vi "Do transition DSP402.vi"(4 "error in (no error)":errorcluster, 6 "State":T1, 7 "DSP402 in":refnum<class "DSP402.lvclass">) -> (0 "error out":errorcluster, 3 "DSP402 out":refnum<class "DSP402.lvclass">)   [LabVIEW 2017, in "canopen.lvlib" / "DSP402.lvclass"]
uses:
  DSP402.lvclass
  DriveState.ctl
  DSP402.lvclass/DSP402.ctl
  types/threestateFlag.ctl
  canopen.lvlib
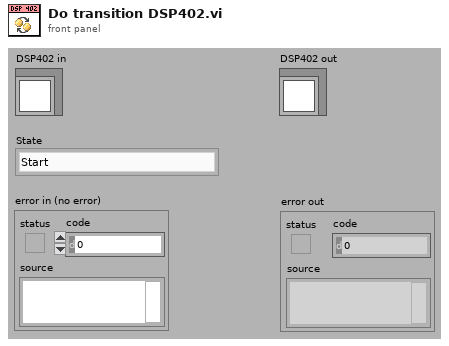
[diagram p1: front panel]
types:
  T1 = typedef "canopen.lvlib/DSP402.lvclass/DriveState.ctl" = enum16{"Start", "Not ready to switch on", "Switch on disabled", "Ready to switch on", "Switched on", "Operation enable", "Fault reaction active", "Fault", "Quick stop active"}
  T2 = typedef "canopen.lvlib/threestateFlag.ctl" = i8
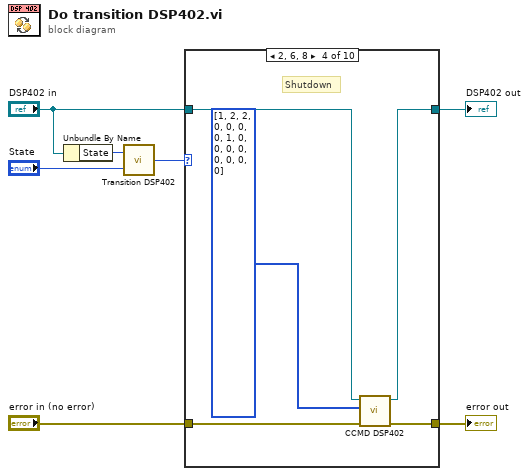
[diagram p0: block diagram]
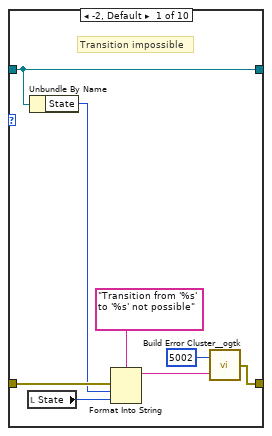
[diagram p2: hidden frame]
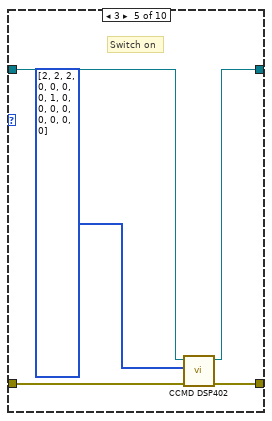
[diagram p5: hidden frame]
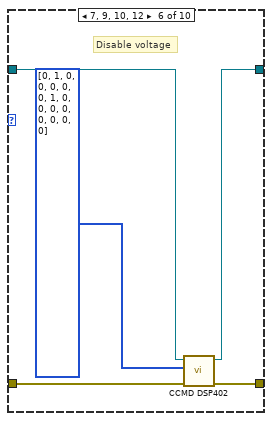
[diagram p6: hidden frame]
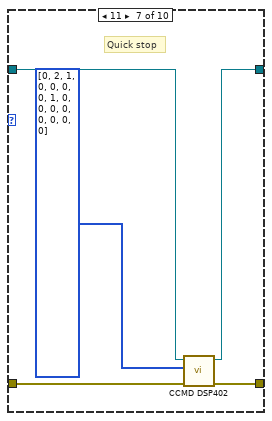
[diagram p7: hidden frame]
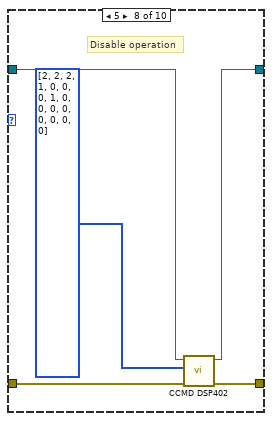
[diagram p8: hidden frame]
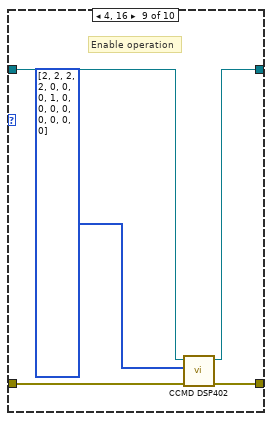
[diagram p9: hidden frame]
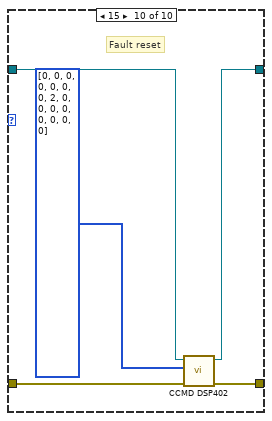
[diagram p10: hidden frame]
diagram:
  n1 = Unbundle By Name("DSP402 in") -> ("State"=w1:T1)
  n2 = call "Transition DSP402.vi"("New state"="State", "Old state"=w1) -> ("Transition"=w3:i32)
  n3 = case shown="2, 6, 8" w3 {
    tunnel: "error in (no error)" -> [w11 w17 w19 w24 w29 w34 w39 w44 w49 w54]
    tunnel: [w13 w17 w19 w23 w28 w33 w38 w43 w48 w53] -> w6
    tunnel: "DSP402 in" -> [w9 w16 w18 w22 w27 w32 w37 w42 w47 w52]
    tunnel: [w9 w16 w18 w21 w26 w31 w36 w41 w46 w51] -> w5
    frame -2, Default {
      # "Transition impossible"
      n4 = local read "State"() -> (w10:T1)
      n5 = Unbundle By Name(w9) -> ("State"=w8:T1)
      n6 = Format Into String(format string="Transition from '%s' to '%s' not possible", error in=w11, w8, w10) -> (resulting string=w12:string)  [unwired: 1 in, 1 out]
      n7 = call <userlib>:"Build Error Cluster__ogtk.vi"("String to Prepend to source (\"\")"=w12, "code"=5002) -> ("error out"=w13:errorcluster)
    }
    frame -1 {
      # "No transition required"
    }
    frame 0, 1, 13, 14 {
      # "Automatic transition"
    }
    frame 2, 6, 8 {
      w20 = T2[] [1, 2, 2, 0, 0, 0, 0, 1, 0, 0, 0, 0, 0, 0, 0, 0] items=["---", "OFF", "ON"] ("Mask")
      # "Shutdown"
      n8 = call "CCMD DSP402.vi"("error in (no error)"=w24, "Mask"=w20, "DSP402 in"=w22) -> ("error out"=w23:errorcluster, "DSP402 out"=w21:refnum<class "DSP402.lvclass">)  [unwired: 3 out]
    }
    frame 3 {
      w25 = T2[] [2, 2, 2, 0, 0, 0, 0, 1, 0, 0, 0, 0, 0, 0, 0, 0] items=["---", "OFF", "ON"] ("Mask")
      # "Switch on"
      n9 = call "CCMD DSP402.vi"("error in (no error)"=w29, "Mask"=w25, "DSP402 in"=w27) -> ("error out"=w28:errorcluster, "DSP402 out"=w26:refnum<class "DSP402.lvclass">)  [unwired: 3 out]
    }
    frame 7, 9, 10, 12 {
      w30 = T2[] [0, 1, 0, 0, 0, 0, 0, 1, 0, 0, 0, 0, 0, 0, 0, 0] items=["---", "OFF", "ON"] ("Mask")
      # "Disable voltage"
      n10 = call "CCMD DSP402.vi"("error in (no error)"=w34, "Mask"=w30, "DSP402 in"=w32) -> ("error out"=w33:errorcluster, "DSP402 out"=w31:refnum<class "DSP402.lvclass">)  [unwired: 3 out]
    }
    frame 11 {
      w35 = T2[] [0, 2, 1, 0, 0, 0, 0, 1, 0, 0, 0, 0, 0, 0, 0, 0] items=["---", "OFF", "ON"] ("Mask")
      # "Quick stop"
      n11 = call "CCMD DSP402.vi"("error in (no error)"=w39, "Mask"=w35, "DSP402 in"=w37) -> ("error out"=w38:errorcluster, "DSP402 out"=w36:refnum<class "DSP402.lvclass">)  [unwired: 3 out]
    }
    frame 5 {
      w40 = T2[] [2, 2, 2, 1, 0, 0, 0, 1, 0, 0, 0, 0, 0, 0, 0, 0] items=["---", "OFF", "ON"] ("Mask")
      # "Disable operation"
      n12 = call "CCMD DSP402.vi"("error in (no error)"=w44, "Mask"=w40, "DSP402 in"=w42) -> ("error out"=w43:errorcluster, "DSP402 out"=w41:refnum<class "DSP402.lvclass">)  [unwired: 3 out]
    }
    frame 4, 16 {
      w45 = T2[] [2, 2, 2, 2, 0, 0, 0, 1, 0, 0, 0, 0, 0, 0, 0, 0] items=["---", "OFF", "ON"] ("Mask")
      # "Enable operation"
      n13 = call "CCMD DSP402.vi"("error in (no error)"=w49, "Mask"=w45, "DSP402 in"=w47) -> ("error out"=w48:errorcluster, "DSP402 out"=w46:refnum<class "DSP402.lvclass">)  [unwired: 2 in, 1 out]
    }
    frame 15 {
      w50 = T2[] [0, 0, 0, 0, 0, 0, 0, 2, 0, 0, 0, 0, 0, 0, 0, 0] items=["---", "OFF", "ON"] ("Mask")
      # "Fault reset"
      n14 = call "CCMD DSP402.vi"("error in (no error)"=w54, "Mask"=w50, "DSP402 in"=w52) -> ("error out"=w53:errorcluster, "DSP402 out"=w51:refnum<class "DSP402.lvclass">)  [unwired: 3 out]
    }
  }
  "error out" <- w6
  "DSP402 out" <- w5
